vi "Read Correct Data.vi"(11 "DataName":string) -> (3 "DataOut":string)   [LabVIEW 2019]
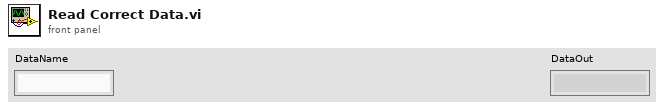
[diagram p1: front panel]
types:
  T1 = enum16{"Initial", "Write", "Read", "Save", "Load", "WrteAll"}
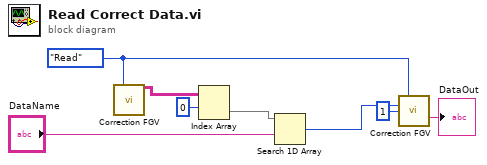
[diagram p0: block diagram]
diagram:
  w4 = T1."Read" ("Action")
  n1 = call "Correction FGV.vi"("Action"=w4) -> ("TableOut"=w8:string[][])  [unwired: 12 in, 2 out]
  n2 = Index Array(array=w8, index (row)=0) -> (element=w6:string[])  [unwired: 1 in]
  n3 = Search 1D Array(1D array=w6, element="DataName") -> (index of element=w3:i32)  [unwired: 1 in]
  n4 = call "Correction FGV.vi"("Action"=w4, "X"=w3, "Y"=1) -> ("DataOut"=→"DataOut":string)  [unwired: 10 in, 2 out]
